vi "BMI160_Temperature.vi"(1 "Word (string, big endian)":string="\u0000\u0000") -> (0 "T (deg C)":sgl=23.0)   [LabVIEW 2015]
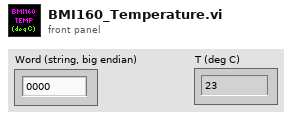
[diagram p1: front panel]
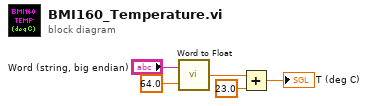
[diagram p0: block diagram]
diagram:
  n1 = call "Word to Float.vi"("Range"=sgl 64.0, "Word (string, big endian)"="Word (string, big endian)") -> ("float32 out"=w3:sgl)
  n2 = Add(x=w3, y=sgl 23.0) -> (x+y=→"T (deg C)":sgl)
